vi "arrays.vi"(3 "Array 3":T1(array[cluster])=[{"Cluster"={"Boolean"=TRUE, "Boolean 2"=FALSE}, "Boolean"=TRUE, "Cluster 2"={"Numeric Control"=2.0}}, {"Cluster"={"Boolean"=FALSE, "Boolean 2"=TRUE}, "Boolean"=FALSE, "Cluster 2"={"Numeric Control"=-1.0}}, {"Cluster"={"Boolean"=FALSE, "Boolean 2"=FALSE}, "Boolean"=TRUE, "Cluster 2"={"Numeric Control"=0.0}}], 4 "Array 2":string[](array[string])=["abc", "def", "ghi", "jkl"], 5 "Array":T2(array[cluster])=[{"Numeric"=1.0, "Horizontal Progress Bar"=41, "Array"=[[[TRUE, TRUE, FALSE, FALSE, FALSE, TRUE, FALSE], [FALSE, TRUE, TRUE, FALSE, TRUE, FALSE, FALSE], [FALSE, FALSE, FALSE, TRUE, FALSE, FALSE, FALSE]]], "Waveform Graph"=[], "XY Graph"=[]}, {"Numeric"=5.0, "Horizontal Progress Bar"=67, "Array"=[[[TRUE, FALSE, TRUE, FALSE, TRUE, FALSE, TRUE], [TRUE, FALSE, TRUE, FALSE, TRUE, FALSE, TRUE], [TRUE, FALSE, TRUE, FALSE, TRUE, FALSE, TRUE]]], "Waveform Graph"=[], "XY Graph"=[]}] {"Horizontal Progress Bar" scale=0.0..100.0}) -> ()   [LabVIEW 2011]
panel:
  out "xml string":string
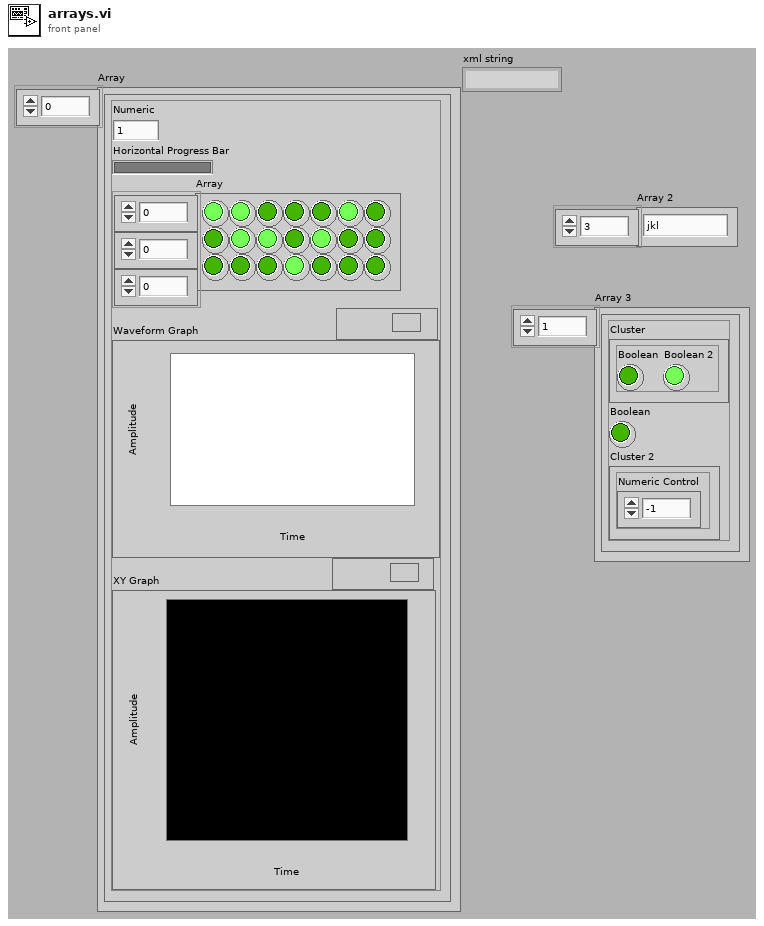
[diagram p1: front panel]
types:
  T1 = cluster{"Cluster":cluster{"Boolean":bool, "Boolean 2":bool}, "Boolean":bool, "Cluster 2":cluster{"Numeric Control":dbl}}[]
  T2 = cluster{"Numeric":dbl, "Horizontal Progress Bar":u8, "Array":bool[][][], "Waveform Graph":dbl[], "XY Graph":cluster{dbl, dbl}[]}[]
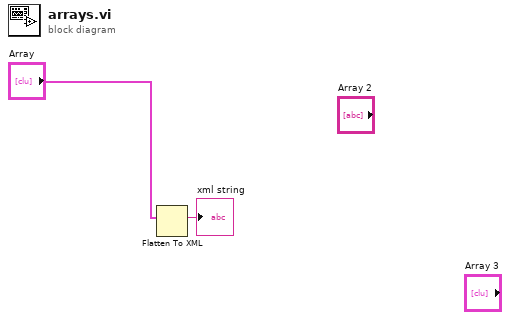
[diagram p0: block diagram]
diagram:
  n1 = Flatten To XML(anything="Array") -> (xml string=→"xml string":string)
